vi "Get Ball Pose.vi"(11 "Detection Ball":T2) -> (3 "Pose":T1)   [LabVIEW 2016]
uses:
  SSL Detection Ball.ctl
  <vilib>/Analysis/Matrix/Datatypes/RealMatrix.ctl
  <vilib>/Analysis/Matrix/Numeric/Conversions/Array To Matrix - RA.vi
  <vilib>/Analysis/Matrix/NI_Matrix.lvlib
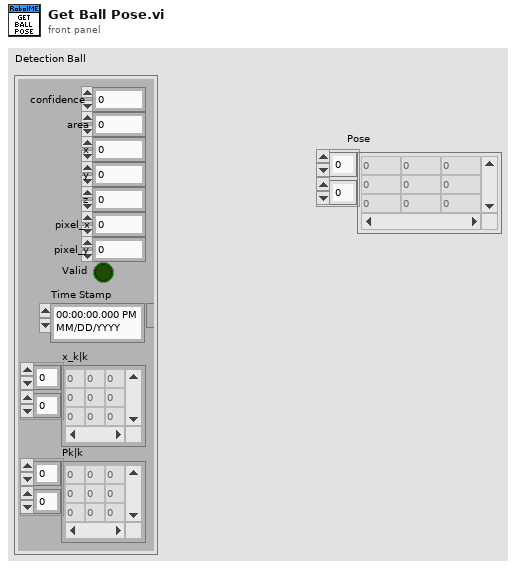
[diagram p1: front panel]
types:
  T1 = typedef "NI_Matrix.lvlib/RealMatrix.ctl" = dbl[][]
  T2 = typedef "SSL Detection Ball.ctl" = cluster{"x":sgl, "area":u32, "confidence":sgl, "y":sgl, "z":sgl, "pixel_x":sgl, "pixel_y":sgl, "Valid":bool, "Time Stamp":timestamp, "x_k|k":T1, "Pk|k":T1}
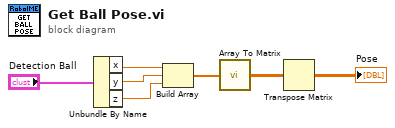
[diagram p0: block diagram]
diagram:
  n1 = Unbundle By Name("Detection Ball") -> ("x"=w5:sgl, "y"=w6:sgl, "z"=w7:sgl)
  n2 = Build Array(w5, w6, w7) -> (w3:sgl[])
  n3 = call-poly <vilib>:"Array To Matrix.vi"("Real 1D Array"=w3) -> ("Real Matrix (Column Vector)"=w2:T1)
  n4 = Transpose Matrix(1:w2) -> (0:→"Pose":T1)
